vi "Get Active Item.vi"(8 "error in (no error)":errorcluster, 11 "Debug Log View In":refnum<class "Debug Log View.lvclass">) -> (0 "error out":errorcluster, 2 "Debug Data":T1, 3 "Debug Log View Out":refnum<class "Debug Log View.lvclass">)   [LabVIEW 2020, in "Debug Log View.lvclass"]
uses:
  Debug Log View.lvclass
  Debugger/TypeDefs/Debug Data.ctl
  Debugger/Debugger.lvclass
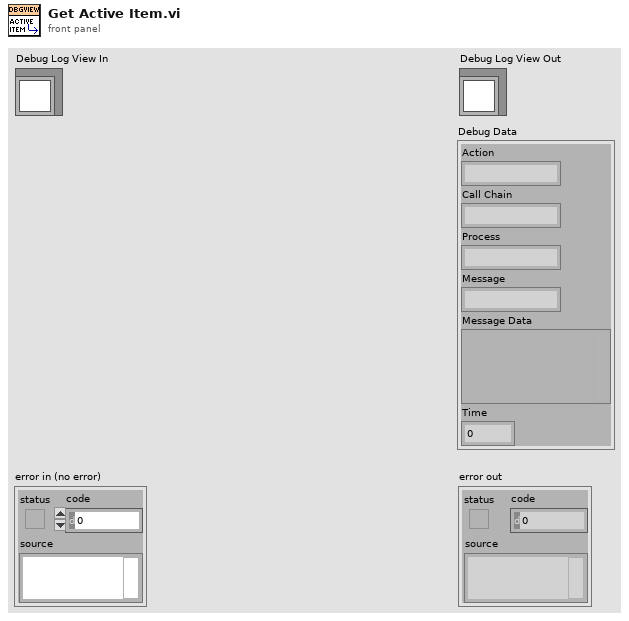
[diagram p1: front panel]
types:
  T1 = typedef "Debugger.lvclass/Debug Data.ctl" = cluster{"Action":string, "Call Chain":string, "Process":string, "Message":string, "Message Data":variant, "Time":u32}
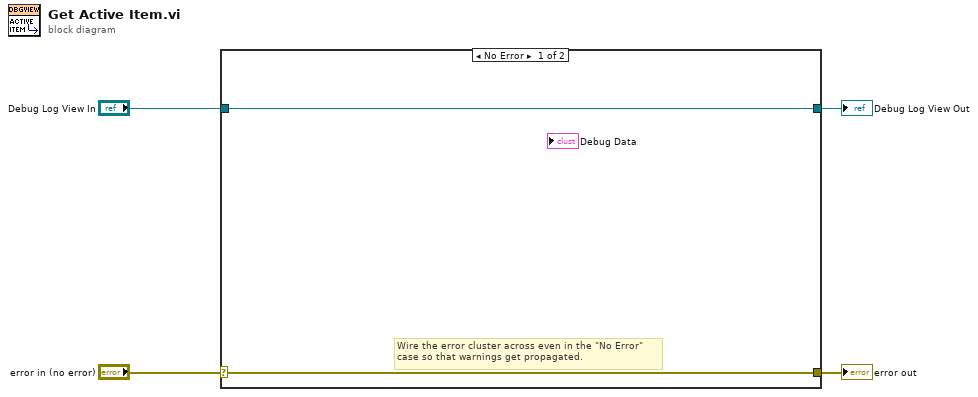
[diagram p0: block diagram]
diagram:
  n1 = case shown="No Error" "error in (no error)" {
    selector: "error in (no error)" -> [w5 w8]
    tunnel: [w5 w8] -> w3
    tunnel: [w6 w7] -> w1
    tunnel: "Debug Log View In" -> [w6 w7]
    frame No Error {
      # "Wire the error cluster across even in the \"No Error\"\ncase so that warnings get propagated."
    }
    frame Error {
    }
  }
  "error out" <- w3
  "Debug Log View Out" <- w1
